vi "Do.vi"(8 "error in (no error)":errorcluster, 10 "Actor in":refnum<class "Actor.lvclass">, 11 "VI Operation Msg":refnum<class "VI Operation Msg.lvclass">) -> (0 "error out":errorcluster, 2 "Actor out":refnum<class "Actor.lvclass">)   [LabVIEW 2015, in "Model.lvlib" / "VI Operation Msg.lvclass"]
doc: "This VI delivers the message to the actor by calling the appropriate method(s) on the actor."
uses:
  VI Operation Msg.lvclass
  Model/Model.lvclass
  Interface Messages/RTM Activated Msg/RTM Activated Msg.lvclass
  <vilib>/ActorFramework/Actor/Actor.lvclass
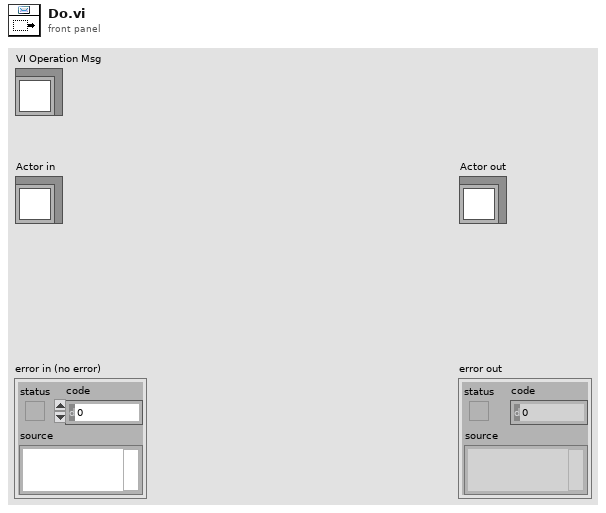
[diagram p1: front panel]
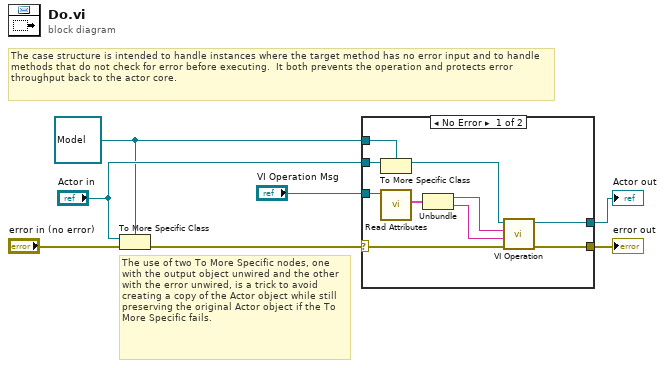
[diagram p0: block diagram]
diagram:
  w2 = refnum<class "Model.lvclass"> refnum ("Actor in")
  # "The use of two To More Specific nodes, one with the output object unwired and the other with the error unwired, is a trick to avoid creating a copy of the Actor object while still preserving the original Actor object if the To More Specific fails."
  # "The case structure is intended to handle instances where the target method has no error input and to handle methods that do not check for error before executing.  It both prevents the operation and protects error throughput back to the actor core."
  n1 = To More Specific Class(target class=w2, reference="Actor in", error in="error in (no error)") -> (error out=w6:errorcluster)  [unwired: 1 out]
  n2 = case shown="No Error" w6 {
    selector: w6 -> [w15 w19]
    tunnel: [w17 w19] -> w5
    tunnel: [w16 w18] -> w4
    tunnel: "Actor in" -> [w14 w18]
    tunnel: w2 -> [w13 _]
    tunnel: "VI Operation Msg" -> [w10 _]
    frame No Error {
      n3 = To More Specific Class(target class=w13, reference=w14) -> (specific class reference=w12:refnum<class "Model.lvclass">)  [unwired: 1 in, 1 out]
      n4 = call "Read Attributes.vi"("RTM Activated Msg"=w10) -> ("Payload"=w11:cluster{"Tag":string, "VI Name":string})  [unwired: 10 in]
      n5 = Unbundle(w11) -> ("Tag"=w8:string, "VI Name"=w9:string)
      n6 = call-dynamic "VI Operation.vi"("error in (no error)"=w15, "VI Name"=w9, "Operation"=w8, "Model in"=w12) -> ("error out"=w17:errorcluster, "Model out"=w16:refnum<class "Model.lvclass">)  [unwired: 6 in]
    }
    frame Error {
      # "If type check fails, pass the original object out again."
    }
  }
  "error out" <- w5
  "Actor out" <- w4
